vi "Configure Trigger (Logic).vi"(0 "VISA resource name":refnum<visa-resource-name>, 1 "Pattern Input":T1={"Channel 1 Logic Input (2: X)"=2, "Channel 2 Logic Input (2: X)"=2, "Channel 3 Logic Input (2: X)"=2, "Channel 4 Logic Input (2: X)"=2, "RF Channel Logic Input (2: X)"=2} {"RF Channel Logic Input (2: X)" items=["High", "Low", "X"]; "Channel 4 Logic Input (2: X)" items=["High", "Low", "X"]; "Channel 3 Logic Input (2: X)" items=["High", "Low", "X"]; "Channel 2 Logic Input (2: X)" items=["High", "Low", "X"]; "Channel 1 Logic Input (2: X)" items=["High", "Low", "X"]}, 2 "RF Logic Threshold (-22dBm)":dbl=-22.0 min=-40.0 max=10.0 step=1.0 format="%#_g dBm", 5 "Function (0: AND)":u16(ring) items=["AND", "OR", "NAND", "NOR"], 7 "Clock Source (1: Channel 1)":u16(ring)=1 items=["None", "Channel 1", "Channel 2", "Channel 3", "Channel 4", "Digital Channel 0", "Digital Channel 1", "Digital Channel 2", "Digital Channel 3", "Digital Channel 4", "Digital Channel 5", "Digital Channel 6", "Digital Channel 7", "Digital Channel 8", "Digital Channel 9", "Digital Channel 10", "Digital Channel 11", "Digital Channel 12", "Digital Channel 13", "Digital Channel 14", "Digital Channel 15", "RF"], 9 "Clock Polarity (0: Rising)":u16(ring) items=["Rising", "Falling"], 11 "error in (no error)":errorcluster, 12 "Trigger Condition (0: True)":u16(ring) items=["True", "False", "Less Than", "More Than", "Equal", "Not Equal"], 13 "Delta Time (4.0ns)":dbl=4e-09) -> (4 "VISA resource name out":refnum<visa-resource-name>, 15 "error out":errorcluster)   [LabVIEW 2017, in "Scope.lvlib" / "Tektronix DPO MSO 2000 4000 Series.lvlib"]
doc: "Configures logic trigger settings for an oscilloscope."
uses:
  Tektronix DPO MSO 2000 4000 Series.lvlib
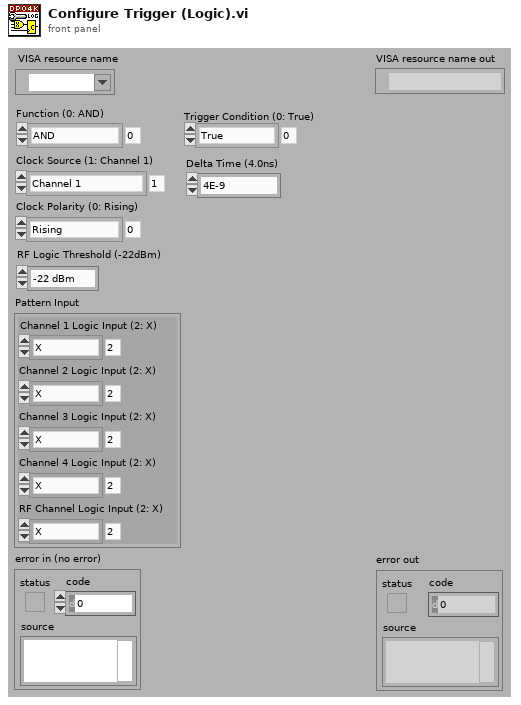
[diagram p1: front panel]
types:
  T1 = cluster{"Channel 1 Logic Input (2: X)":u16, "Channel 2 Logic Input (2: X)":u16, "Channel 3 Logic Input (2: X)":u16, "Channel 4 Logic Input (2: X)":u16, "RF Channel Logic Input (2: X)":u16}
  T2 = typedef "Scope.lvlib/Tektronix DPO MSO 2000 4000 Series.lvlib/Extended User Data.ctl" = cluster{"DPO MSO Series Model":u16}
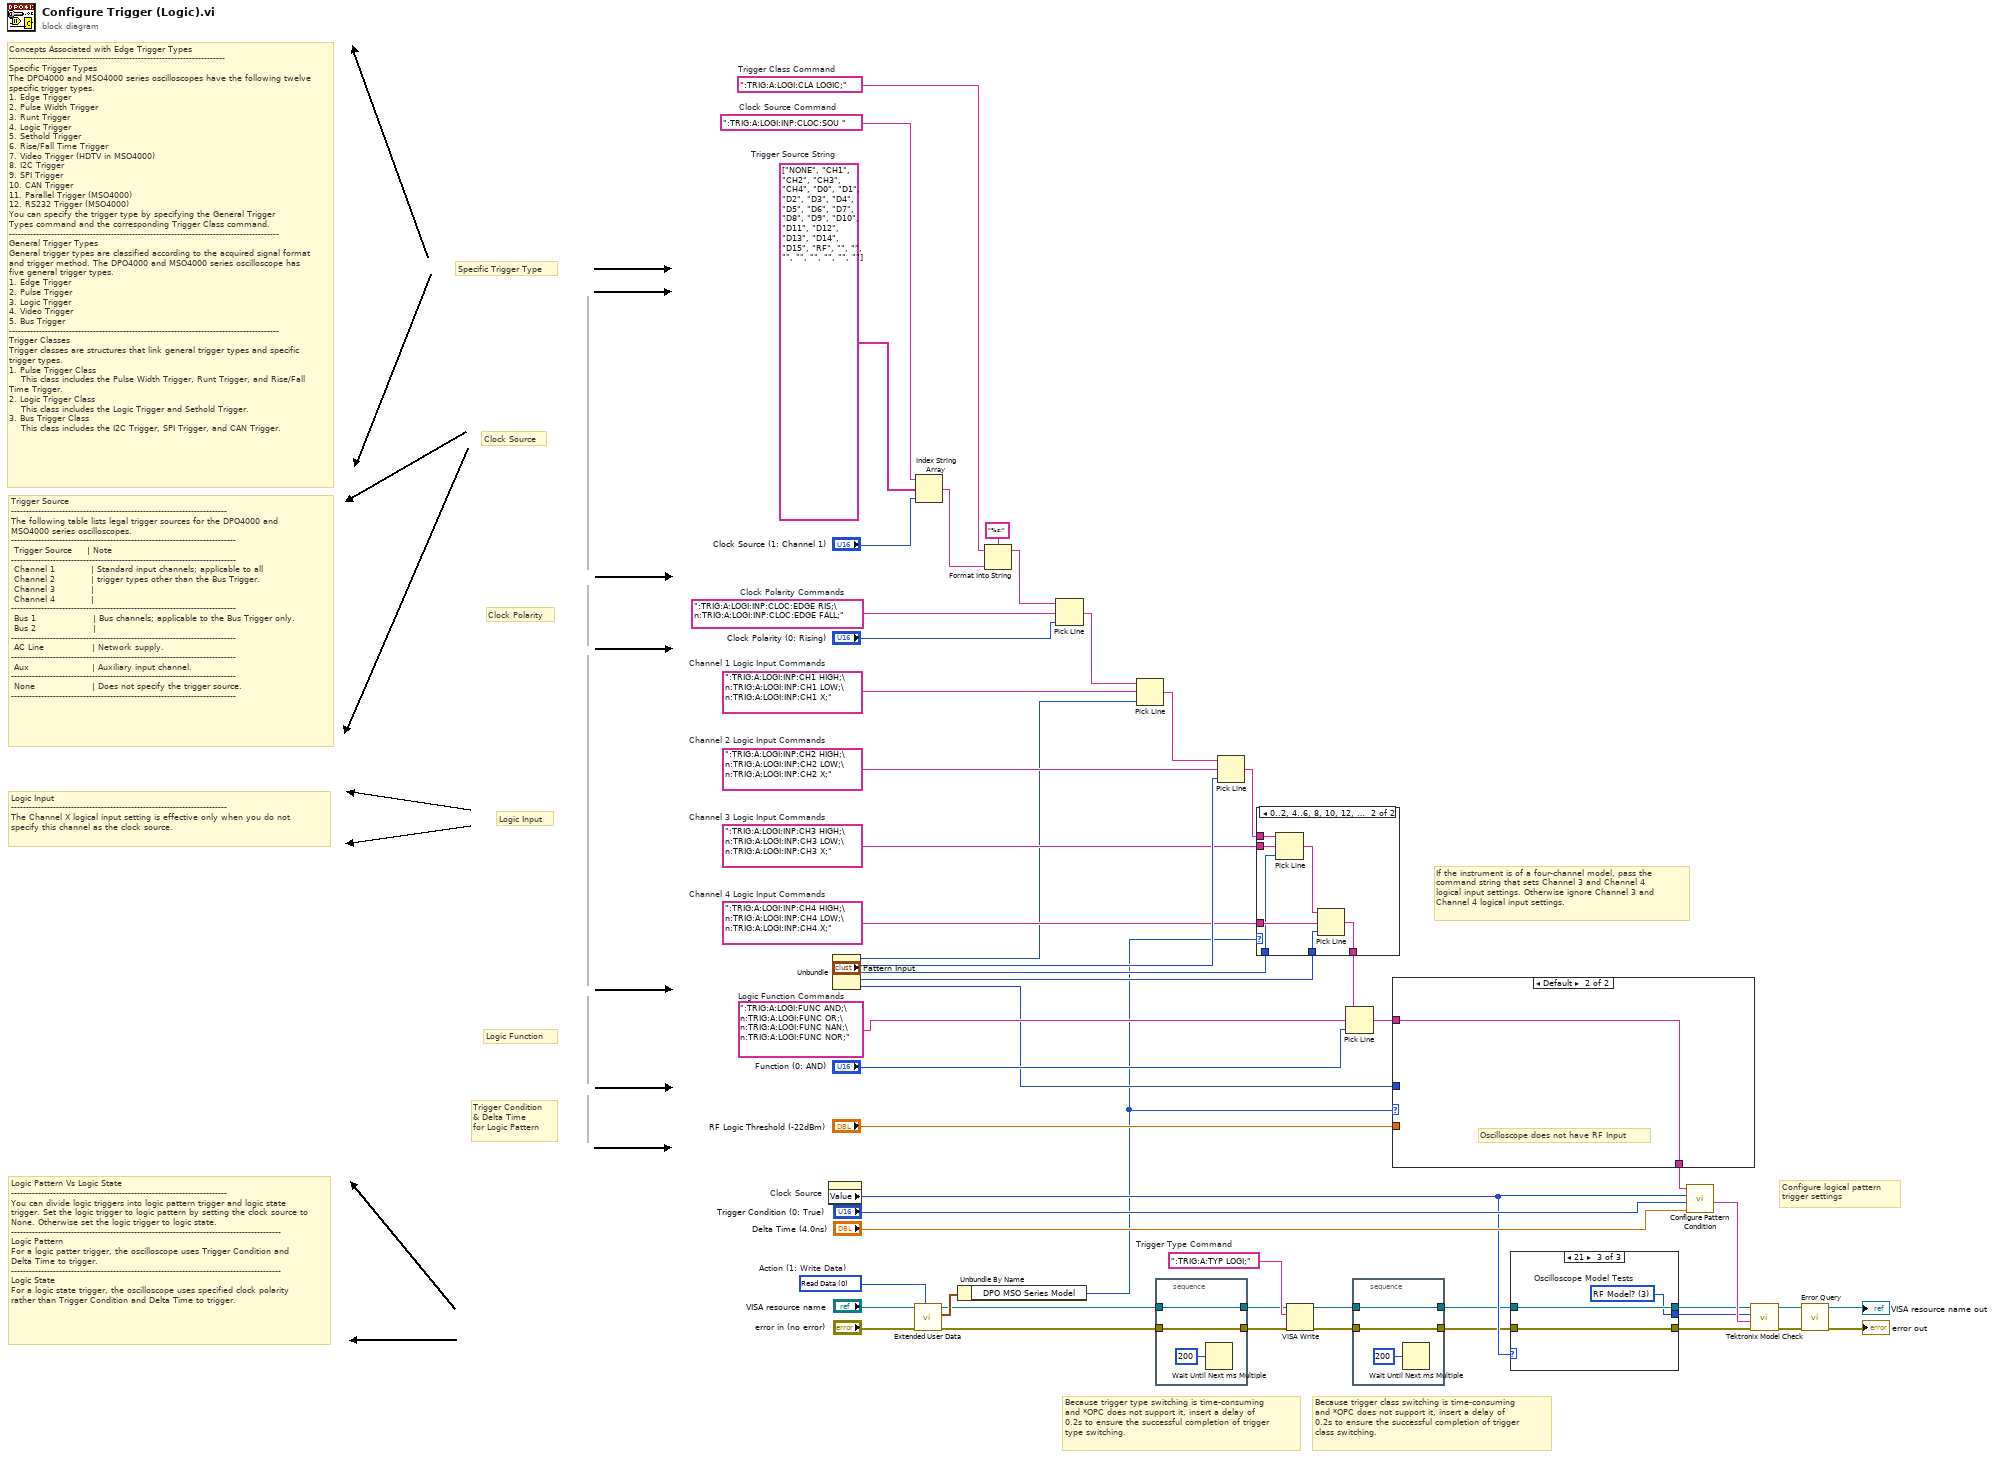
[diagram p0: block diagram]
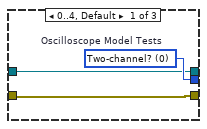
[diagram p2: hidden frame]
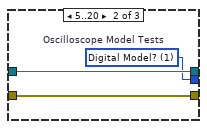
[diagram p3: hidden frame]
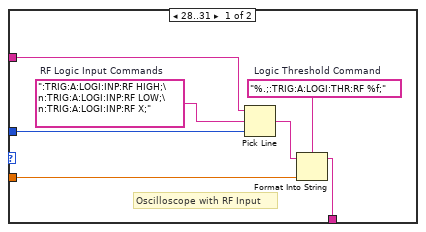
[diagram p4: hidden frame]
diagram:
  w6 = 0 items=["Read Data", "Write Data", "Clear Data", "Clear ALL Data"]  # Action (1: Write Data)
  w27 = string[] ["NONE", "CH1", "CH2", "CH3", "CH4", "D0", "D1", "D2", "D3", "D4", "D5", "D6", "D7", "D8", "D9", "D10", "D11", "D12", "D13", "D14", "D15", "RF", "", "", "", "", "", "", "", ""]  # Trigger Source String
  w37 = ":TRIG:A:LOGI:INP:CH4 HIGH;\n:TRIG:A:LOGI:INP:CH4 LOW;\n:TRIG:A:LOGI:INP:CH4 X;"  # Channel 4 Logic Input Commands
  w38 = ":TRIG:A:LOGI:INP:CH3 HIGH;\n:TRIG:A:LOGI:INP:CH3 LOW;\n:TRIG:A:LOGI:INP:CH3 X;"  # Channel 3 Logic Input Commands
  w42 = ":TRIG:A:LOGI:INP:CH2 HIGH;\n:TRIG:A:LOGI:INP:CH2 LOW;\n:TRIG:A:LOGI:INP:CH2 X;"  # Channel 2 Logic Input Commands
  w43 = ":TRIG:A:LOGI:INP:CH1 HIGH;\n:TRIG:A:LOGI:INP:CH1 LOW;\n:TRIG:A:LOGI:INP:CH1 X;"  # Channel 1 Logic Input Commands
  w46 = ":TRIG:A:LOGI:FUNC AND;\n:TRIG:A:LOGI:FUNC OR;\n:TRIG:A:LOGI:FUNC NAN;\n:TRIG:A:LOGI:FUNC NOR;"  # Logic Function Commands
  w48 = ":TRIG:A:LOGI:INP:CLOC:EDGE RIS;\n:TRIG:A:LOGI:INP:CLOC:EDGE FALL;"  # Clock Polarity Commands
  w50 = ":TRIG:A:LOGI:INP:CLOC:SOU "  # Clock Source Command
  w26 = ":TRIG:A:LOGI:CLA LOGIC;"  # Trigger Class Command
  w53 = ":TRIG:A:TYP LOGI;"  # Trigger Type Command
  # "Trigger Source\n------------------------------------------------------------------------\nThe following table lists legal trigger sources for the DPO4000 and MSO4000 series oscilloscopes.\n---------------------------------------------------------------------------\n Trigger Source     | Note                                                           \n---------------------------------------------------------------------------\n Channel 1            | Standard input channels; applicable to all      \n Channel 2            | trigger types other than the Bus Trigger.         \n Channel 3            |     \n Channel 4            |\n---------------------------------------------------------------------------\n Bus 1                   | Bus channels; applicable to the Bus Trigger only.\n Bus 2                   | \n---------------------------------------------------------------------------\n AC Line                | Network supply.\n---------------------------------------------------------------------------\n Aux                     | Auxiliary input channel.\n---------------------------------------------------------------------------\n None                   | Does not specify the trigger source.\n---------------------------------------------------------------------------"
  # "Concepts Associated with Edge Trigger Types\n------------------------------------------------------------------------\nSpecific Trigger Types\nThe DPO4000 and MSO4000 series oscilloscopes have the following twelve specific trigger types.\n1. Edge Trigger\n2. Pulse Width Trigger\n3. Runt Trigger\n4. Logic Trigger\n5. Sethold Trigger\n6. Rise/Fall Time Trigger\n7. Video Trigger (HDTV in MSO4000)\n8. I2C Trigger\n9. SPI Trigger\n10. CAN Trigger\n11. Parallel Trigger (MSO4000)\n12. RS232 Trigger (MSO4000)\nYou can specify the trigger type by specifying the General Trigger \nTypes command and the corresponding Trigger Class command.\n------------------------------------------------------------------------------------------\nGeneral Trigger Types \nGeneral trigger types are classified according to the acquired signal format and trigger method. The DPO4000 and MSO4000 series oscilloscope has five general trigger types.\n1. Edge Trigger\n2. Pulse Trigger\n3. Logic Trigger\n4. Video Trigger\n5. Bus Trigger\n------------------------------------------------------------------------------------------\nTrigger Classes\nTrigger classes are structures that link general trigger types and specific trigger types.\n1. Pulse Trigger Class\n    This class includes the Pulse Width Trigger, Runt Trigger, and Rise/Fall Time Trigger.\n2. Logic Trigger Class\n    This class includes the Logic Trigger and Sethold Trigger.\n3. Bus Trigger Class\n    This class includes the I2C Trigger, SPI Trigger, and CAN Trigger."
  # "Because trigger type switching is time-consuming\nand *OPC does not support it, insert a delay of\n0.2s to ensure the successful completion of trigger\ntype switching."
  # "Because trigger class switching is time-consuming\nand *OPC does not support it, insert a delay of\n0.2s to ensure the successful completion of trigger\nclass switching."
  # "Configure logical pattern\ntrigger settings"
  # "If the instrument is of a four-channel model, pass the\ncommand string that sets Channel 3 and Channel 4\nlogical input settings. Otherwise ignore Channel 3 and\nChannel 4 logical input settings."
  # "Logic Pattern Vs Logic State\n------------------------------------------------------------------------\nYou can divide logic triggers into logic pattern trigger and logic state trigger. Set the logic trigger to logic pattern by setting the clock source to None. Otherwise set the logic trigger to logic state.\n------------------------------------------------------------------------------------------\nLogic Pattern\nFor a logic patter trigger, the oscilloscope uses Trigger Condition and Delta Time to trigger.\n------------------------------------------------------------------------------------------\nLogic State\nFor a logic state trigger, the oscilloscope uses specified clock polarity rather than Trigger Condition and Delta Time to trigger."
  # "Logic Input\n------------------------------------------------------------------------\nThe Channel X logical input setting is effective only when you do not specify this channel as the clock source."
  # "Trigger Condition\n& Delta Time \nfor Logic Pattern"
  # "Logic Function"
  # "Logic Input"
  # "Clock Polarity"
  # "Clock Source"
  # "Specific Trigger Type"
  n1 = property on="Clock Source" class="Ring (strict)"() -> ("Value"=w13:u16)  [unwired: 2 in, 2 out]
  n2 = Unbundle("Pattern Input") -> ("Channel 1 Logic Input (2: X)"=w22:u16, "Channel 2 Logic Input (2: X)"=w40:u16, "Channel 3 Logic Input (2: X)"=w36:u16, "Channel 4 Logic Input (2: X)"=w35:u16, "RF Channel Logic Input (2: X)"=w16:u16)
  n3 = call "Extended User Data.vi"("Action (1: Write Data)"=w6, "error in (no error)"="error in (no error)", "VISA resource name"="VISA resource name") -> ("error out"=w1:errorcluster, "User Data Out"=w7:T2, "VISA resource name out"=w2:refnum<visa-resource-name>)  [unwired: 6 in]
  n4 = Index String Array(1:"Clock Source (1: Channel 1)", 2:w27, 3:w50) -> (0:w25:string)
  n5 = Unbundle By Name(w7) -> ("DPO MSO Series Model"=w5:u16)
  n6 = Format Into String(format string="%s;", initial string=w26, w25) -> (resulting string=w47:string)  [unwired: 1 in, 1 out]
  n7 = Pick Line(string ("")=w47, multi-line string=w48, line index="Clock Polarity (0: Rising)") -> (output string=w24:string)
  n8 = Pick Line(string ("")=w24, multi-line string=w43, line index=w22) -> (output string=w41:string)
  n9 = stacked-sequence {
    tunnel: w2 -> [w55]
    tunnel: [w55] -> w52
    tunnel: w1 -> [w54]
    tunnel: [w54] -> w51
    frame #0 {
      n10 = Wait Until Next ms Multiple(millisecond multiple=u32 200) -> ()  [unwired: 1 out]
    }
  }
  n11 = Pick Line(string ("")=w41, multi-line string=w42, line index=w40) -> (output string=w39:string)
  n12 = case shown="0..2, 4..6, 8, 10, 12, 15, 17, 19..21, 24, 25, 69..73" w5 {
    tunnel: w39 -> [w57 w64]
    tunnel: w38 -> [_ w63]
    tunnel: w37 -> [_ w61]
    tunnel: w36 -> [_ w60]
    tunnel: w35 -> [_ w59]
    tunnel: [w57 w58] -> w23
    frame 3, 7, 9, 11, 13, 14, 16, 18, 22, 23, 26, 27, Default {
    }
    frame 0..2, 4..6, 8, 10, 12, 15, 17, 19..21, 24, 25, 69..73 {
      n13 = Pick Line(string ("")=w64, multi-line string=w63, line index=w60) -> (output string=w62:string)
      n14 = Pick Line(string ("")=w62, multi-line string=w61, line index=w59) -> (output string=w58:string)
    }
  }
  n15 = VISA Write(VISA resource name=w52, write buffer=w53, error in (no error)=w51) -> (VISA resource name out=w34:refnum<visa-resource-name>, error out=w33:errorcluster)  [unwired: 1 out]
  n16 = Pick Line(string ("")=w23, multi-line string=w46, line index="Function (0: AND)") -> (output string=w17:string)
  n17 = stacked-sequence {
    tunnel: w34 -> [w66]
    tunnel: [w66] -> w12
    tunnel: w33 -> [w65]
    tunnel: [w65] -> w10
    frame #0 {
      n18 = Wait Until Next ms Multiple(millisecond multiple=u32 200) -> ()  [unwired: 1 out]
    }
  }
  n19 = case shown="Default" w5 {
    tunnel: w17 -> [w72 w75]
    tunnel: w16 -> [w73 _]
    tunnel: "RF Logic Threshold (-22dBm)" -> [w71 _]
    tunnel: [w68 w75] -> w14
    frame 28..31 {
      w69 = "%.;:TRIG:A:LOGI:THR:RF %f;"  # Logic Threshold Command
      w74 = ":TRIG:A:LOGI:INP:RF HIGH;\n:TRIG:A:LOGI:INP:RF LOW;\n:TRIG:A:LOGI:INP:RF X;"  # RF Logic Input Commands
      # "Oscilloscope with RF Input"
      n20 = Pick Line(string ("")=w72, multi-line string=w74, line index=w73) -> (output string=w70:string)
      n21 = Format Into String(format string=w69, initial string=w70, w71) -> (resulting string=w68:string)  [unwired: 1 in, 1 out]
    }
    frame Default {
      # "Oscilloscope does not have RF Input"
    }
  }
  n22 = case shown="21" w13 {
    tunnel: w12 -> [w76 w81 w84]
    tunnel: [w76 w81 w84] -> w11
    tunnel: w10 -> [w77 w80 w83]
    tunnel: [w77 w80 w83] -> w9
    tunnel: [w78 w79 w82] -> w8
    frame 0..4, Default {
      w78 = u16 0 items=["Two-channel?", "Digital Model?", "Four-channel?", "RF Model?"]  # Oscilloscope Model Tests
    }
    frame 5..20 {
      w79 = u16 1 items=["Two-channel?", "Digital Model?", "Four-channel?", "RF Model?"]  # Oscilloscope Model Tests
    }
    frame 21 {
      w82 = u16 3 items=["Two-channel?", "Digital Model?", "Four-channel?", "RF Model?"]  # Oscilloscope Model Tests
    }
  }
  n23 = call "Configure Pattern Condition.vi"("Delta Time (2.5E-9)"="Delta Time (4.0ns)", "Trigger Condition (0: True)"="Trigger Condition (0: True)", "Clock Source (0: Channel 1)"=w13, "Input Command String"=w14) -> ("Output Command String"=w20:string)  [unwired: 7 in]
  n24 = call "Tektronix Model Check.vi"("error in (no error)"=w9, "Command String"=w20, "Oscilloscope Model Tests (3: RF Model?)"=w8, "VISA resource name"=w11) -> ("error out"=w18:errorcluster, "VISA resource name out"=w19:refnum<visa-resource-name>)  [unwired: 6 in]
  n25 = call "Error Query.vi"("error in (no error)"=w18, "VISA resource name"=w19) -> ("error out"=→"error out":errorcluster, "VISA resource name out"=→"VISA resource name out":refnum<visa-resource-name>)  [unwired: 6 in, 2 out]
